vi "Teleop.vi"(10 "Match Info":T1={"Autonomous Elapsed Seconds"=0.0, "TeleOp Elapsed Seconds"=0.0, "Disabled Elapsed Seconds"=0.0, "Visited Autonomous"=FALSE, "Visited TeleOp"=FALSE, "Visited Disabled"=FALSE, "Autonomous Settings"={"Autonomous Style"=enum."Independent", "VI Refnum"=refnum}}, 11 "Call Context":T2) -> ()   [LabVIEW 2017]
doc: "This VI is called for each TeleOp packet received from the DS where the robot is not disabled. It is often used to read from the joysticks and update I/O or to update setpoints for timed control loops. It should complete and return within 20 milliseconds or it may miss DS packets."
uses:
  <vilib>/Rock Robotics/WPI/DriverStation/WPI_DriverStationDerivedRobotMode.ctl
  <vilib>/Rock Robotics/WPI/DriverStation/WPI_DriverStationMatch Info.ctl
  <vilib>/Rock Robotics/WPI/Utilities/WPI_GetSetVariantRefNum.vi
  <vilib>/Rock Robotics/Network Tables/NT Write Boolean Array.vi
  <vilib>/Rock Robotics/Network Tables/NT Write Numeric Array.vi
  <vilib>/Rock Robotics/Network Tables/NT Read Boolean.vi
  <vilib>/Rock Robotics/Network Tables/NT Read Number.vi
panel:
  out "Sample Slider 0":dbl(slide) scale=0.0..5.0
  out "Sample Boolean 1":bool
  out "Sample Boolean 0":bool
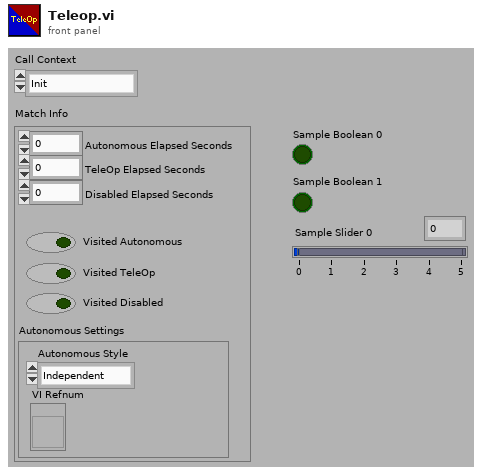
[diagram p1: front panel]
types:
  T1 = typedef "WPI_DriverStationMatch Info.ctl" = cluster{"Autonomous Elapsed Seconds":dbl, "TeleOp Elapsed Seconds":dbl, "Disabled Elapsed Seconds":dbl, "Visited Autonomous":bool, "Visited TeleOp":bool, "Visited Disabled":bool, "Autonomous Settings":cluster{"Autonomous Style":enum16{"Iterative", "Independent"}, "VI Refnum":refnum<vi>}}
  T2 = typedef "WPI_DriverStationDerivedRobotMode.ctl" = enum16{"Init", "Execute", "Stop"}
  T3 = typedef "WPI_JoystickDevRef.ctl" = cluster{"Device":T4}
  T4 = typedef "WPI_JoystickDeviceEnum.ctl" = enum16{"USB 0", "USB 1", "USB 2", "USB 3", "USB 4", "USB 5"}
  T5 = typedef "WPI_RobotDriveDevRef.ctl" = cluster{"DevStatus":errorcluster, "Motors[]":T6[], "Square Inputs":bool, "Max Output":dbl}
  T6 = typedef "WPI_MotorControlDeviceRef.ctl" = cluster{"DeviceStatus":errorcluster, "Type":T7, "PWM":cluster{"PWM Channel":T8, "DeadBand":T9}, "CAN":cluster{"Device Number":u8, "SetOutput VI Ref":variant, "GetOutput VI Ref":variant, "Enable VI Ref":variant, "Disable VI Ref":variant, "Data":variant}, "Invert":bool, "DIO PWM":cluster{"PWM \"Enable\" Channel":T8, "DIOChannel":T10, "PWM Rate":dbl}}
  T7 = typedef "WPI_MotorControlType.ctl" = enum16{"PWM", "CAN", "DIO PWM"}
  T8 = typedef "FPGA_DIOPWMChannel.ctl" = enum8{"PWM 0", "PWM 1", "PWM 2", "PWM 3", "PWM 4", "PWM 5", "PWM 6", "PWM 7", "PWM 8", "PWM 9", "PWM MXP 0", "PWM MXP 1", "PWM MXP 2", "PWM MXP 3", "PWM MXP 4", "PWM MXP 5", "PWM MXP 6", "PWM MXP 7", "PWM MXP 8", "PWM MXP 9", "Invalid"}
  T9 = typedef "WPI_PWMDeadband.ctl" = cluster{"Name":string, "maxPositivePwm":i32, "minPositivePwm":i32, "centerPwm":i32, "maxNegativePwm":i32, "minNegativePwm":i32, "angularRange":u16}
  T10 = typedef "FPGA_DIOChannel.ctl" = enum8{"DIO 0", "DIO 1", "DIO 2", "DIO 3", "DIO 4", "DIO 5", "DIO 6", "DIO 7", "DIO 8", "DIO 9", "DIO MXP 0", "DIO MXP 1", "DIO MXP 2", "DIO MXP 3", "DIO MXP 4", "DIO MXP 5", "DIO MXP 6", "DIO MXP 7", "DIO MXP 8", "DIO MXP 9", "DIO MXP 10", "DIO MXP 11", "DIO MXP 12", "DIO MXP 13", "DIO MXP 14", "DIO MXP 15", "SPI Port CS1", "SPI Port CS2", "SPI Port CS3", "SPI Port MISO", "SPI Port MOSI", "Invalid"}
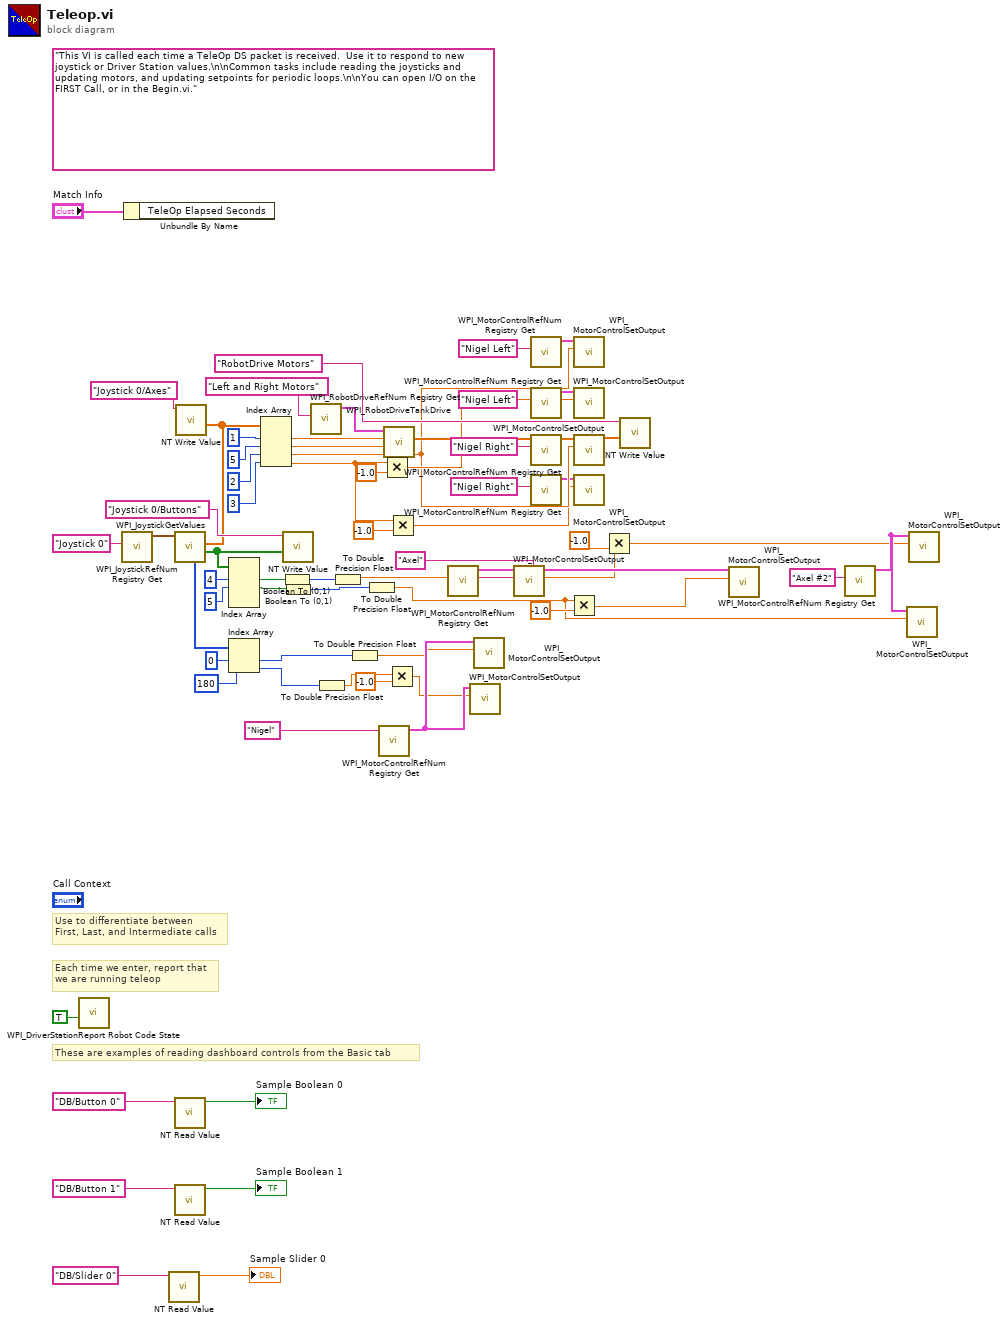
[diagram p0: block diagram]
diagram:
  (unwired) "This VI is called each time a TeleOp DS packet is received.  Use it to respond to new joystick or Driver Station values.\n\nCommon tasks include reading the joysticks and updating motors, and updating setpoints for periodic loops.\n\nYou can open I/O on the FIRST Call, or in the Begin.vi."
  # "These are examples of reading dashboard controls from the Basic tab"
  # "Each time we enter, report that\nwe are running teleop"
  # "Use to differentiate between\nFirst, Last, and Intermediate calls"
  n1 = call <vilib>:"WPI_DriverStationReport Robot Code State.vi"("TeleOp"=TRUE ("Autonomous")) -> ()  [unwired: 10 in, 1 out]
  n2 = call <vilib>:"WPI_JoystickRefNum Registry Get.vi"("refnum name"="Joystick 0") -> ("JoystickDevRef"=w60:T3)  [unwired: 1 in, 9 out]
  n3 = Unbundle By Name("Match Info") -> ()  [unwired: 1 out]
  n4 = call-poly <vilib>:"NT Read Value.vi"("Name"="DB/Slider 0" ("refnum name")) -> ("Numeric"=→"Sample Slider 0":dbl)  [unwired: 9 in, 1 out]
  n5 = call <vilib>:"WPI_JoystickGetValues.vi"("JoystickDevRef"=w60) -> ("Buttons"=w38:bool[], "Axes"=w55:dbl[], "POVs"=w23:i16[])  [unwired: 6 in, 2 out]
  n6 = call-poly <vilib>:"NT Read Value.vi"("Name"="DB/Button 0" ("refnum name")) -> ("Boolean"=→"Sample Boolean 0":bool)  [unwired: 9 in, 1 out]
  n7 = call-poly <vilib>:"NT Read Value.vi"("Name"="DB/Button 1" ("refnum name")) -> ("Boolean"=→"Sample Boolean 1":bool)  [unwired: 9 in, 1 out]
  n8 = call-poly <vilib>:"NT Write Value.vi"("Numeric Array"=w55, "Name"="Joystick 0/Axes") -> ()  [unwired: 9 in, 1 out]
  n9 = Index Array(array=w38, index #1=4 ("index"), index #2=5 ("index")) -> (element #1=w35:bool, element #2=w34:bool)  [unwired: 2 in, 2 out]
  n10 = Index Array(array=w23, index #1=0 ("index"), index #2=180 ("index")) -> (element #1=w20:i16, element #2=w19:i16)
  n11 = Index Array(array=w55, index #1=1 ("index"), index #2=5 ("index"), index #3=2 ("index"), index #4=3 ("index")) -> (element #1=w62:dbl, element #2=w58:dbl, element #3=w27:dbl, element #4=w2:dbl)
  n12 = Boolean To (0,1)(Boolean=w35) -> (0, 1=w33:i16)
  n13 = call-poly <vilib>:"NT Write Value.vi"("Boolean Array"=w38, "Name"="Joystick 0/Buttons") -> ()  [unwired: 9 in, 1 out]
  n14 = Boolean To (0,1)(Boolean=w34) -> (0, 1=w32:i16)
  n15 = call <vilib>:"WPI_RobotDriveRefNum Registry Get.vi"("refnum name"="Left and Right Motors") -> ("RobotDriveDevRef"=w63:T5)  [unwired: 1 in, 9 out]
  n16 = To Double Precision Float(number=w19) -> (double precision float=w16:dbl)
  n17 = To Double Precision Float(number=w33) -> (double precision float=w6:dbl)
  n18 = To Double Precision Float(number=w20) -> (double precision float=w13:dbl)
  n19 = To Double Precision Float(number=w32) -> (double precision float=w3:dbl)
  n20 = call <vilib>:"WPI_MotorControlRefNum Registry Get.vi"("refnum name"="Nigel") -> ("MotorControlDevRef"=w17:T6)  [unwired: 9 in, 1 out]
  n21 = Multiply(x=w2, y=-1.0) -> (x*y=w39:dbl)
  n22 = call <vilib>:"WPI_RobotDriveTankDrive.vi"("Right axis value"=w58, "Left axis value"=w62, "RobotDriveDevRef"=w63) -> ("Motor Values"=w48:dbl[])  [unwired: 6 in, 2 out]
  n23 = Multiply(x=w16, y=-1.0) -> (x*y=w14:dbl)
  n24 = Multiply(x=w2, y=-1.0) -> (x*y=w24:dbl)
  n25 = call <vilib>:"WPI_MotorControlRefNum Registry Get.vi"("refnum name"="Axel") -> ("MotorControlDevRef"=w11:T6)  [unwired: 9 in, 1 out]
  n26 = call <vilib>:"WPI_MotorControlSetOutput.vi"("Output"=w14, "MotorControlDevRef"=w17) -> ()  [unwired: 7 in, 3 out]
  n27 = call <vilib>:"WPI_MotorControlSetOutput.vi"("Output"=w13, "MotorControlDevRef"=w17) -> ()  [unwired: 7 in, 3 out]
  n28 = call <vilib>:"WPI_MotorControlSetOutput.vi"("Output"=w6, "MotorControlDevRef"=w11) -> ()  [unwired: 7 in, 3 out]
  n29 = call <vilib>:"WPI_MotorControlRefNum Registry Get.vi"("refnum name"="Nigel Left") -> ("MotorControlDevRef"=w41:T6)  [unwired: 9 in, 1 out]
  n30 = call <vilib>:"WPI_MotorControlRefNum Registry Get.vi"("refnum name"="Nigel Left") -> ("MotorControlDevRef"=w30:T6)  [unwired: 9 in, 1 out]
  n31 = call <vilib>:"WPI_MotorControlRefNum Registry Get.vi"("refnum name"="Nigel Right") -> ("MotorControlDevRef"=w28:T6)  [unwired: 9 in, 1 out]
  n32 = call <vilib>:"WPI_MotorControlRefNum Registry Get.vi"("refnum name"="Nigel Right") -> ("MotorControlDevRef"=w25:T6)  [unwired: 9 in, 1 out]
  n33 = Multiply(x=w3, y=-1.0) -> (x*y=w4:dbl)
  n34 = call <vilib>:"WPI_MotorControlSetOutput.vi"("Output"=w27, "MotorControlDevRef"=w41) -> ()  [unwired: 7 in, 3 out]
  n35 = call <vilib>:"WPI_MotorControlSetOutput.vi"("Output"=w39, "MotorControlDevRef"=w30) -> ()  [unwired: 7 in, 3 out]
  n36 = call <vilib>:"WPI_MotorControlSetOutput.vi"("Output"=w27, "MotorControlDevRef"=w28) -> ()  [unwired: 7 in, 3 out]
  n37 = call <vilib>:"WPI_MotorControlSetOutput.vi"("Output"=w24, "MotorControlDevRef"=w25) -> ()  [unwired: 7 in, 3 out]
  n38 = Multiply(x=w6, y=-1.0) -> (x*y=w7:dbl)
  n39 = call-poly <vilib>:"NT Write Value.vi"("Numeric Array"=w48, "Name"="RobotDrive Motors") -> ()  [unwired: 9 in, 1 out]
  n40 = call <vilib>:"WPI_MotorControlSetOutput.vi"("Output"=w4, "MotorControlDevRef"=w11) -> ()  [unwired: 7 in, 3 out]
  n41 = call <vilib>:"WPI_MotorControlRefNum Registry Get.vi"("refnum name"="Axel #2") -> ("MotorControlDevRef"=w9:T6)  [unwired: 9 in, 1 out]
  n42 = call <vilib>:"WPI_MotorControlSetOutput.vi"("Output"=w3, "MotorControlDevRef"=w9) -> ()  [unwired: 7 in, 3 out]
  n43 = call <vilib>:"WPI_MotorControlSetOutput.vi"("Output"=w7, "MotorControlDevRef"=w9) -> ()  [unwired: 7 in, 3 out]
